vi "通信状态入队列.vi"(8 "错误输入（无错误）":errorcluster, 11 "枚举":enum16{"打开连接", "发送数据", "读取数据", "数据处理", "关闭连接"}(ring)) -> (0 "错误输出":errorcluster)   [LabVIEW 2016, in "数据传输系统.lvlib"]
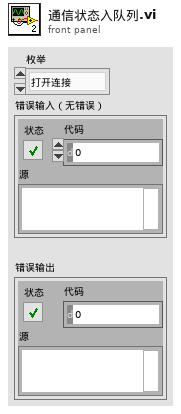
[diagram p1: front panel]
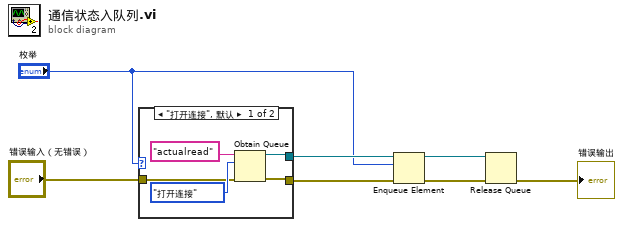
[diagram p0: block diagram]
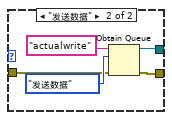
[diagram p2: hidden frame]
diagram:
  n1 = case shown="\"打开连接\", 默认" "枚举" {
    tunnel: [w10 w15] -> w6
    tunnel: [w9 w14] -> w5
    tunnel: "错误输入（无错误）" -> [w8 w13]
    frame "打开连接", Default {
      n2 = Obtain Queue(name (unnamed)="actualread" ("名称（未命名）"), element data type=enum16{"打开连接", "发送数据", "读取数据", "数据处理", "关闭连接"}."打开连接" ("枚举"), error in (no error)=w8) -> (queue out=w10:refnum<queue>, error out=w9:errorcluster)  [unwired: 2 in, 1 out]
    }
    frame "发送数据" {
      n3 = Obtain Queue(name (unnamed)="actualwrite" ("名称（未命名）"), element data type=enum16{"打开连接", "发送数据", "读取数据", "数据处理", "关闭连接"}."发送数据" ("枚举"), error in (no error)=w13) -> (queue out=w15:refnum<queue>, error out=w14:errorcluster)  [unwired: 2 in, 1 out]
    }
  }
  n4 = Enqueue Element(queue=w6, element="枚举", error in (no error)=w5) -> (queue out=w7:refnum<queue>, error out=w4:errorcluster)  [unwired: 1 in, 1 out]
  n5 = Release Queue(queue=w7, error in (no error)=w4) -> (error out=→"错误输出":errorcluster)  [unwired: 1 in, 2 out]
